vi "While Loop With Timeout and Stop Button.vi"() -> ()   [LabVIEW 2017]
doc: "Use this VI as a template. This VI is a simple while structure that shows the interation times with a stop control button."
panel:
  out "indicator":i32
  in  "stop":bool
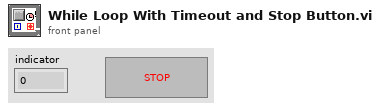
[diagram p1: front panel]
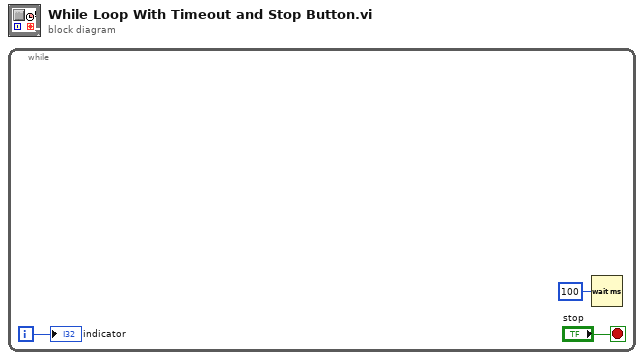
[diagram p0: block diagram]
diagram:
  n1 = while {
    i -> [w1]
    stop <- "stop" stop-if-true
    n2 = Wait (ms)(milliseconds to wait=u32 100) -> ()  [unwired: 1 out]
    "indicator" <- w1
  }
